vi "configure.vi"(8 "error in (no error)":errorcluster, 11 "DL090602SutterMP285Stage in":refnum<class "StageMH100301DMC.lvclass">) -> (0 "error out":errorcluster, 3 "DL090602SutterMP285Stage out":refnum<class "StageMH100301DMC.lvclass">)   [LabVIEW 2010, in "StageMH100301DMC.lvclass"]
doc: "The dynamic dispatch version of this VI loads and displays the configuration file associated with the plug-in object. The user modify and save the configuration data."
uses:
  StageMH100301DMC.lvclass
  StageMH100301DMC.lvclass/StageMH100301DMC.ctl
  common/classes/GenericComponent/GenericComponent/GenericComponent.lvclass
panel:
  in  "Speed (x/y/z)":dbl[unit][](array[numeric])=[0.0, 0.0, 0.0]
  in  "Step factors (x/y/z) (cts/um)":dbl[unit][](array[numeric])=[0.0, 0.0, 0.0]
  out "Configuration":string
  in  "cancel button":bool
  in  "save button":bool
  in  "Serial port name":refnum<visa-resource-name>
  # "Configure MH100301DMC"
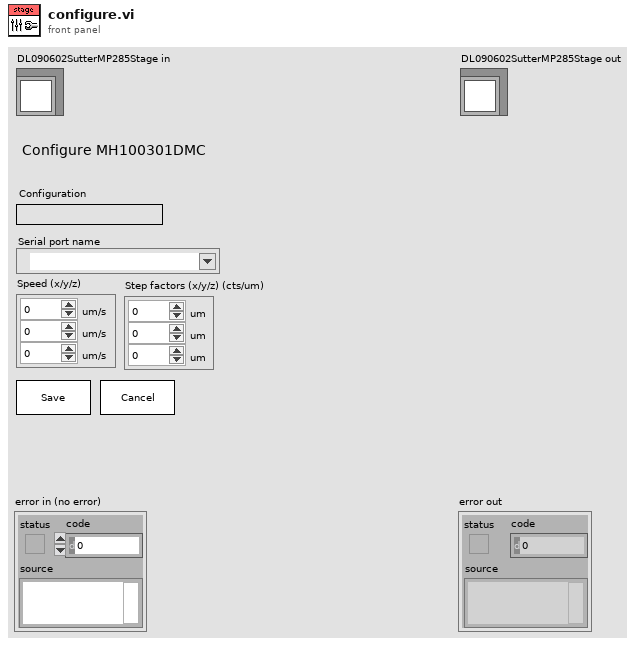
[diagram p1: front panel]
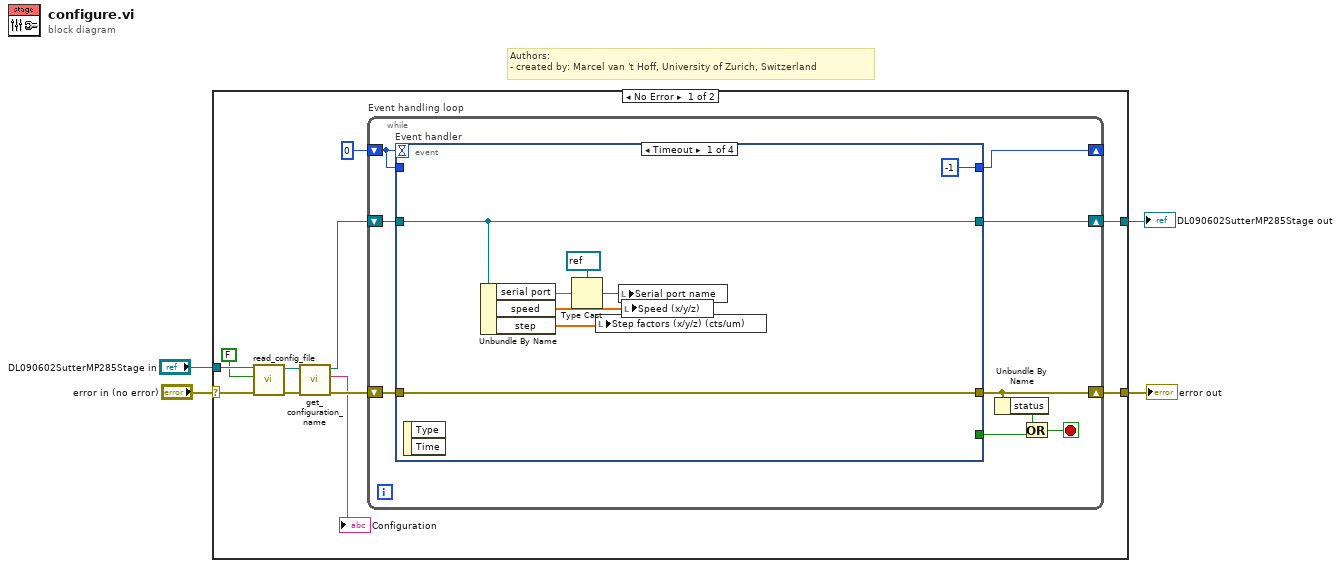
[diagram p0: block diagram]
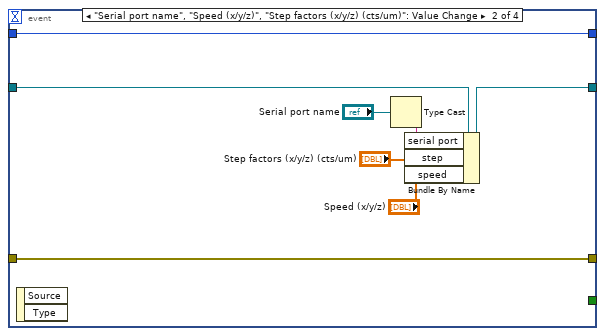
[diagram p2: hidden frame]
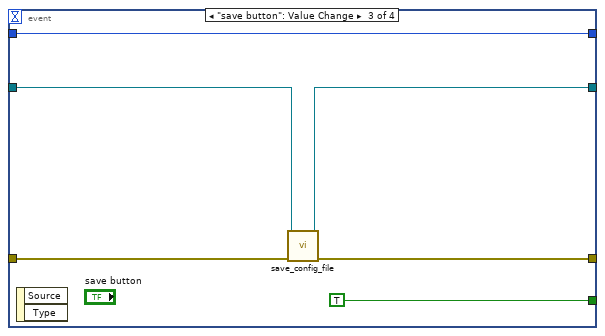
[diagram p3: hidden frame]
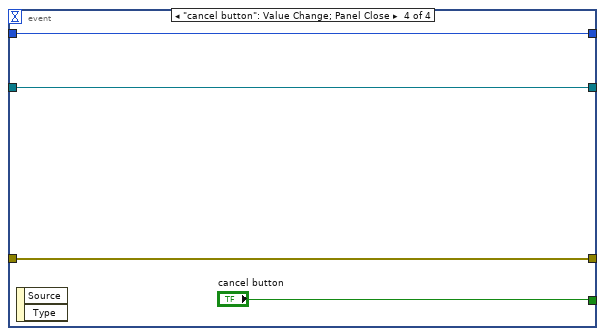
[diagram p4: hidden frame]
diagram:
  # "Authors: \n- created by: Marcel van 't Hoff, University of Zurich, Switzerland"
  n1 = case shown="No Error" "error in (no error)" {
    selector: "error in (no error)" -> [w12 w52]
    tunnel: [w15 w52] -> w3
    tunnel: "DL090602SutterMP285Stage in" -> [w11 w51]
    tunnel: [w14 w51] -> w1
    frame No Error {
      n2 = call-dynamic "read_config_file.vi"("error in (no error)"=w12, "force load?"=FALSE, "GenericPlugin in"=w11) -> ("error out"=w9:errorcluster, "GenericPlugin out"=w7:refnum<class "StageMH100301DMC.lvclass">)  [unwired: 7 out]
      n3 = call "get_configuration_name.vi"("error in (no error)"=w9, "GenericPlugin.lvclass in"=w7) -> ("error out"=w8:errorcluster, "configuration name"=→"Configuration":string, "GenericPlugin.lvclass out"=w6:refnum<class "StageMH100301DMC.lvclass">)  [unwired: 7 in]
      n4 = while "Event handling loop" {
        shift-right: [w19] -> w15
        shift-left: w8 -> [w24]
        shift-right: [w22] -> w14
        shift-left: w6 -> [w23]
        shift-right: [w20] -> _
        shift-left: 0 -> [w21]
        stop <- w16 stop-if-true
        n5 = event "Event handler" shown="[0] Timeout" {
          selector: _ -> [_ _ _ _]
          dyn-events: _ -> [_ _ _ _]
          timeout: w21 -> [_ _ _ _]
          tunnel: w24 -> [w32 w36 w44 w50]
          tunnel: w23 -> [w30 w35 w42 w49]
          tunnel: [w32 w36 w43 w50] -> w19
          tunnel: [w30 w38 w41 w49] -> w22
          tunnel: [-1 w40 w46 w48] -> w20
          tunnel: w21 -> [_ w40 w46 w48]
          tunnel: [_ _ TRUE "cancel button"] -> w18
          event Timeout {
            n6 = event-data() -> ()  [unwired: 3 out]
            n7 = Unbundle By Name(w30) -> ("serial port"=w29:string, "speed"=w25:dbl[unit][], "step"=w26:dbl[unit][])
            n8 = Type Cast(type=refnum<visa-resource-name> refnum ("Serial port name"), x=w29) -> (*(type *) &x=w28:refnum<visa-resource-name>)
            n9 = local write "Step factors (x/y/z) (cts/um)"(w26) -> ()
            n10 = local write "Serial port name"(w28) -> ()
            n11 = local write "Speed (x/y/z)"(w25) -> ()
          }
          event "Serial port name", "Speed (x/y/z)", "Step factors (x/y/z) (cts/um)": Value Change {
            n12 = event-data() -> ()  [unwired: 3 out]
            n13 = Type Cast(x="Serial port name") -> (*(type *) &x=w37:string)  [unwired: 1 out]
            n14 = Bundle By Name(cluster=w35, "serial port"=w37, "step"="Step factors (x/y/z) (cts/um)", "speed"="Speed (x/y/z)") -> (w38:refnum<class "StageMH100301DMC.lvclass">)
          }
          event "save button": Value Change {
            n15 = event-data() -> ()  [unwired: 3 out]
            n16 = call-dynamic "save_config_file.vi"("error in (no error)"=w44, "GenericPlugin in"=w42) -> ("error out"=w43:errorcluster, "GenericPlugin out"=w41:refnum<class "StageMH100301DMC.lvclass">)  [unwired: 1 in, 7 out]
          }
          event "cancel button": Value Change; Panel Close {
            n17 = event-data() -> ()  [unwired: 3 out]
          }
        }
        n18 = Unbundle By Name(w19) -> ("status"=w17:bool)
        n19 = Or(x=w17, y=w18) -> (x .or. y?=w16:bool)
      }
    }
    frame Error {
    }
  }
  "error out" <- w3
  "DL090602SutterMP285Stage out" <- w1
